vi "Set Dwell Time.vi"(8 "Error In":errorcluster caption="Error", 9 "Dwell time":dbl[unit]=0.5 format="%#_1g", 10 "Set # Periods":bool, 11 "VISA resource name":refnum<visa-resource-name>="GPIB0::23::INSTR") -> (0 "Error Out":errorcluster, 3 "VISA resource name out":refnum<visa-resource-name>="GPIB0::23::INSTR")   [LabVIEW 2015, in "SR400.lvlib"]
uses:
  SR400.lvlib
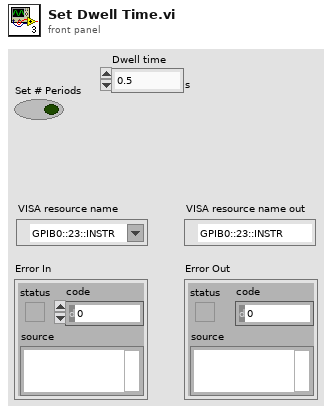
[diagram p1: front panel]
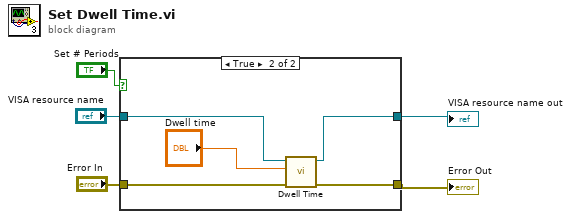
[diagram p0: block diagram]
diagram:
  n1 = case shown="True" "Set # Periods" {
    tunnel: "Error In" -> [w7 w11]
    tunnel: [w7 w9] -> w2
    tunnel: "VISA resource name" -> [w6 w12]
    tunnel: [w6 w10] -> w1
    frame False {
    }
    frame True {
      n2 = call "Dwell Time.vi"("error in (no error)"=w11, "Dwell time (0.002 s)"="Dwell time", "VISA resource name"=w12) -> ("error out"=w9:errorcluster, "VISA resource name out"=w10:refnum<visa-resource-name>)  [unwired: 7 in]
    }
  }
  "Error Out" <- w2
  "VISA resource name out" <- w1
